vi "EditOptions.vi"(8 "error in":errorcluster, 11 "Engine in":refnum<class "Engine Parent Editor Node.lvclass">) -> (0 "error out":errorcluster, 1 "edit options":T1, 2 "subnodes class":T2, 3 "Engine out":refnum<class "Engine Parent Editor Node.lvclass">)   [LabVIEW 2013, in "PL Framework Configuration Tool.lvlib" / "Engine Parent Editor Node.lvclass"]
doc: "This VI Contains the options for the Menu that will be displayed when doing right click on an item\nThe subnodes class configures which nodes can be added to this nodes\nAnd the edit options determine which options are available for the node.\n\nThis configuration is stored in this VI in case some dynamic configuration is required for the menu options or subnodes.\n\nAll VIs must overide this method"
uses:
  Engine Parent Editor Node.lvclass
  <vilib>/NI/Configuration Framework/Node/SubNodeCluster.ctl
  <vilib>/NI/Configuration Framework/Node/NodeMenuOptions.ctl
  Targets/Targets.lvclass
  <vilib>/NI/Configuration Framework/Node/NISE_CEF_Node.lvclass/NISE_CEF_Node.ctl
  Module editor node/module editor node.lvclass
  Framework Configuration Classes/target configuration/PL_Target Configuration.lvclass/PL_Target Configuration.ctl
  Framework Configuration Classes/class cache/cache data.vi
  <vilib>/NI/Configuration Framework/Node/NISE_CEF_Node.lvclass
  Framework Configuration Classes/class cache/PL_class cache.lvlib
  Framework Configuration Classes/target configuration/PL_Target Configuration.lvclass
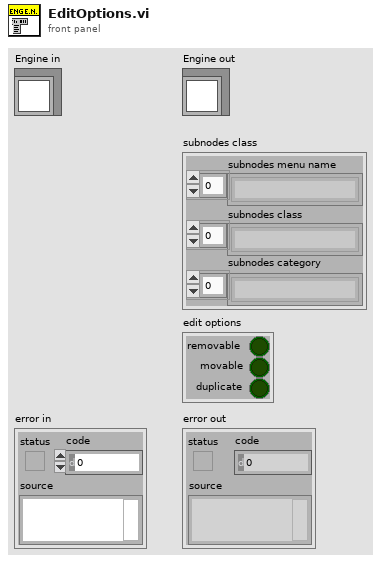
[diagram p1: front panel]
types:
  T1 = typedef "NISE_CEF_Node.lvclass/NodeMenuOptions.ctl" = cluster{"removable":bool, "movable":bool, "duplicate":bool}
  T2 = typedef "NISE_CEF_Node.lvclass/SubNodeCluster.ctl" = cluster{"subnodes menu name":string[], "subnodes class":string[], "subnodes category":string[]}
  T3 = typedef "NISE_CEF_Node.lvclass/NodeRef.ctl" = refnum<data-value>
  T4 = typedef "TBM configuration.lvclass/Target Types.ctl" = enum16{"Windows", "Mac", "Linux", "Linux RT ARM", "VxWorks", "Pharlap", "Other", "Linux RT x64"}
  T5 = typedef "PL_class cache.lvlib/cached class information.ctl" = cluster{"targets":T6[], "engines":T7[], "modules":T7[], "ignored class list":path[]}
  T6 = typedef "PL_class cache.lvlib/target class metadata.ctl" = cluster{"file name":string, "fully qualified name":string, "menu display name":string, "configuration class name":string}
  T7 = typedef "PL_class cache.lvlib/class metadata.ctl" = cluster{"file name":string, "fully qualified name":string, "menu display name":string, "configuration class":string, "category":string, "instances allowed":i32, "supported targets":T4[]}
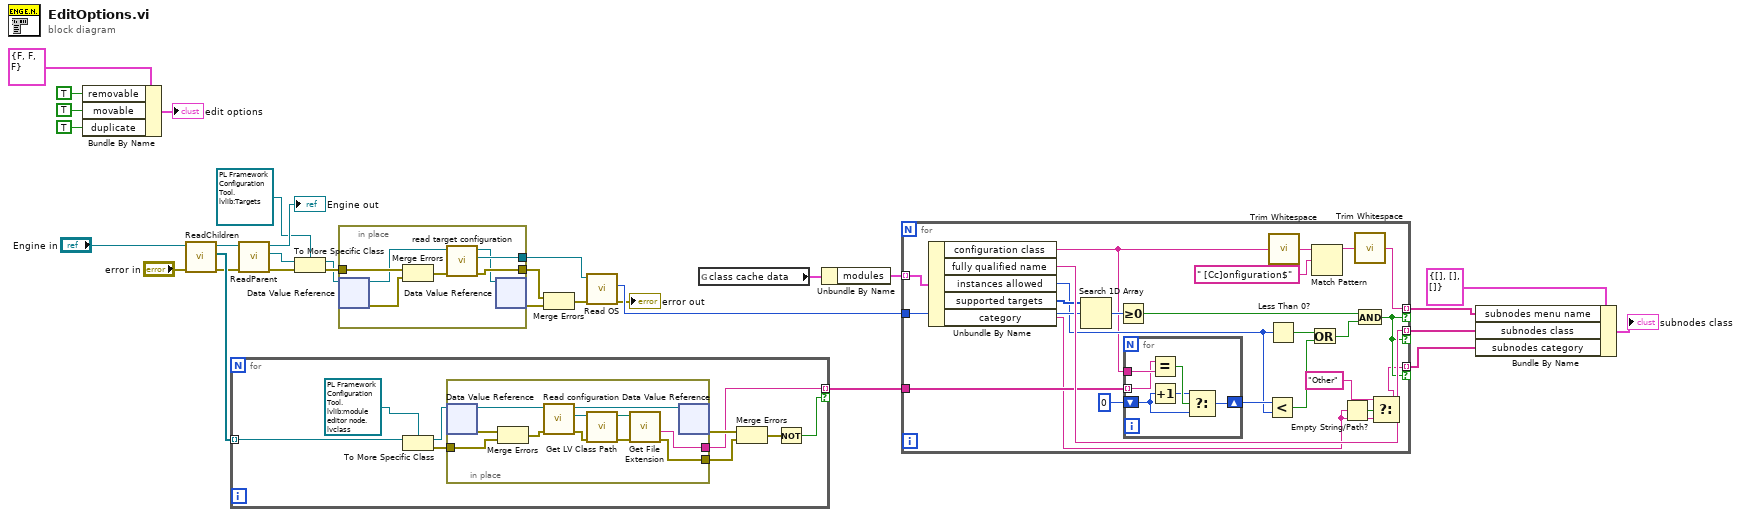
[diagram p0: block diagram]
diagram:
  n1 = Bundle By Name(cluster=T1 {"removable"=FALSE, "movable"=FALSE, "duplicate"=FALSE} ("edit options"), "removable"=TRUE, "movable"=TRUE, "duplicate"=TRUE) -> (→"edit options":T1)
  n2 = call <vilib>:"ReadChildren.vi"("error in"="error in", "node in"="Engine in") -> ("error out"=w10:errorcluster, "output array"=w21:T3[], "node out"=w11:refnum<class "Engine Parent Editor Node.lvclass">)  [unwired: 7 in]
  n3 = for {
    tunnel: w21 -> [w39] mode=indexing
    tunnel: [w31] -> w20 mode=indexing if=w32
    n4 = To More Specific Class(target class=refnum<data-value> refnum, reference=w39) -> (specific class reference=w37:refnum<data-value>, error out=w36:errorcluster)  [unwired: 1 in]
    n5 = in-place {
      in-place-border: w36 -> [w49]
      in-place-border: [w44] -> w31
      in-place-border: [w43] -> w34
      n6 = in-place-dvr #1(w37) -> (w42:refnum<class "module editor node.lvclass">, w50:errorcluster)
      n7 = Merge Errors(w50, w49) -> (w41:errorcluster)
      n8 = call-dynamic "Read configuration.vi"("error in"=w41, "NISE_CEF_serializable node in"=w42) -> ("error out"=w47:errorcluster, "configuration"=w45:refnum<class "NISE_CEF_serializable configuration.lvclass">, "NISE_CEF_serializable node out"=w40:refnum<class "module editor node.lvclass">)  [unwired: 7 in]
      n9 = call <vilib>:"Get LV Class Path.vi"("error in (no error)"=w47, "object"=w45) -> ("error out"=w46:errorcluster, "class path"=w48:path)  [unwired: 8 in]
      n10 = call <vilib>:"Get File Extension.vi"("error in (no error)"=w46, "file"=w48) -> ("error out"=w43:errorcluster, "filename without extension"=w44:string)  [unwired: 6 in, 2 out]
      n11 = in-place-dvr #1(w40) -> (w35:errorcluster)  [unwired: 1 out]
    }
    n12 = Merge Errors(w35, w34) -> (w33:errorcluster)
    n13 = Not(x=w33) -> (.not. x?=w32:bool)
  }
  n14 = call <vilib>:"ReadParent.vi"("error in"=w10, "node in"=w11) -> ("error out"=w6:errorcluster, "parent"=w7:T3, "node out"=→"Engine out":refnum<class "Engine Parent Editor Node.lvclass">)  [unwired: 7 in]
  n15 = To More Specific Class(target class=refnum<data-value> refnum, reference=w7, error in=w6) -> (specific class reference=w4:refnum<data-value>, error out=w5:errorcluster)
  n16 = in-place {
    in-place-border: [w57] -> w15
    in-place-border: [w56] -> w14
    in-place-border: w5 -> [w55]
    n17 = in-place-dvr #2(w4) -> (w54:refnum<class "Targets.lvclass">, w51:errorcluster)
    n18 = Merge Errors(w55, w51) -> (w52:errorcluster)
    n19 = call "read target configuration.vi"("error in"=w52, "Targets in"=w54) -> ("error out"=w57:errorcluster, "Target Configuration"=w56:refnum<class "PL_Target Configuration.lvclass">, "Targets out"=w53:refnum<class "Targets.lvclass">)  [unwired: 7 in]
    n20 = in-place-dvr #2(w53) -> (w2:errorcluster)  [unwired: 1 out]
  }
  n21 = Merge Errors(w15, w2) -> (w3:errorcluster)
  n22 = call "Read OS.vi"("error in"=w3, "PL_Target Configuration in"=w14) -> ("error out"=→"error out":errorcluster, "Target Types"=w13:T4)  [unwired: 7 in, 1 out]
  n23 = global read "cache data.vi" "class cache data"() -> (w23:T5)
  n24 = Unbundle By Name(w23) -> ("modules"=w22:T7[])
  n25 = for {
    tunnel: w22 -> [w80] mode=indexing
    tunnel: [w63] -> w17 mode=indexing if=w62
    tunnel: [w79] -> w16 mode=indexing if=w62
    tunnel: w20 -> [w75]
    tunnel: w13 -> [w77]
    tunnel: [w58] -> w1 mode=indexing if=w62
    n26 = Unbundle By Name(w80) -> ("configuration class"=w64:string, "fully qualified name"=w79:string, "instances allowed"=w69:i32, "supported targets"=w78:T4[], "category"=w60:string)
    n27 = Search 1D Array(1D array=w78, element=w77) -> (index of element=w76:i32)  [unwired: 1 in]
    n28 = Greater Or Equal To 0?(x=w76) -> (x >= 0?=w71:bool)
    n29 = for {
      tunnel: w75 -> [w85] mode=indexing
      tunnel: w64 -> [w86]
      shift-right: [w81] -> w73
      shift-left: 0 -> [w82]
      n30 = Equal?(x=w85, y=w86) -> (x = y?=w84:bool)
      n31 = Increment(x=w82) -> (x+1=w83:i32)
      n32 = Select(t=w83, s=w84, f=w82) -> (s? t:f=w81:i32)
    }
    n33 = Less?(x=w73, y=w69) -> (x < y?=w72:bool)
    n34 = Less Than 0?(x=w69) -> (x < 0?=w68:bool)
    n35 = call <vilib>:"Trim Whitespace.vi"("string"=w64) -> ("trimmed string"=w65:string)  [unwired: 1 in]
    n36 = Or(x=w68, y=w72) -> (x .or. y?=w70:bool)
    n37 = Match Pattern(string=w65, regular expression=" [Cc]onfiguration$") -> (before substring=w67:string)  [unwired: 1 in, 3 out]
    n38 = Empty String/Path?(string/path=w60) -> (empty?=w61:bool)
    n39 = call <vilib>:"Trim Whitespace.vi"("string"=w67) -> ("trimmed string"=w63:string)  [unwired: 1 in]
    n40 = And(x=w71, y=w70) -> (x .and. y?=w62:bool)
    n41 = Select(t="Other", s=w61, f=w60) -> (s? t:f=w58:string)
  }
  n42 = Bundle By Name(cluster=T2 {"subnodes menu name"=[], "subnodes class"=[], "subnodes category"=[]} ("subnodes class"), "subnodes menu name"=w17, "subnodes class"=w16, "subnodes category"=w1) -> (→"subnodes class":T2)
